vi "Result Step Measure Meter Reading query.vi"(8 "error in (no error)":errorcluster, 10 "Step":T1=1 min=1 max=99 step=1, 11 "VISA resource name":refnum<visa-resource-name>) -> (0 "error out":errorcluster, 2 "Result":string, 3 "VISA resource name out":refnum<visa-resource-name>)   [LabVIEW 2025]
uses:
  <instrlib>/Chroma 19052/Public/Utility/Type Def/steps--numeric.ctl
  <instrlib>/Chroma 19052/Chroma 19052.lvlib
panel:
  # "Step Measure Meter Reading"
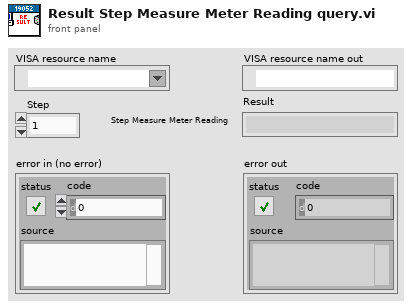
[diagram p1: front panel]
types:
  T1 = typedef "Chroma 19052.lvlib/steps--numeric.ctl" = u8
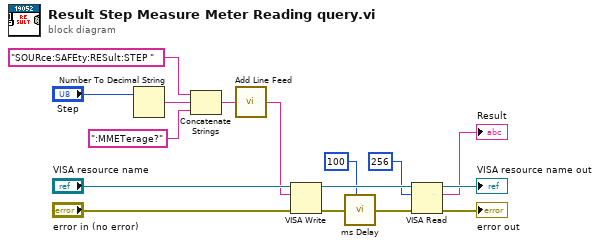
[diagram p0: block diagram]
diagram:
  n1 = Number To Decimal String(number="Step") -> (decimal integer string=w6:string)  [unwired: 1 in]
  n2 = Concatenate Strings("SOURce:SAFEty:RESult:STEP ", w6, ":MMETerage?") -> (w3:string)
  n3 = call <instrlib>:"Add Line Feed.vi"("Command string"=w3) -> ("Concatenated string"=w10:string)  [unwired: 4 in]
  n4 = VISA Write(VISA resource name="VISA resource name", write buffer=w10, error in (no error)="error in (no error)") -> (VISA resource name out=w16:refnum<visa-resource-name>, error out=w15:errorcluster)  [unwired: 1 out]
  n5 = call <instrlib>:"ms Delay.vi"("miliseconds to wait"=u32 100 ("Time Delay ms"), "error in (no error)"=w15) -> ("error out"=w14:errorcluster)  [unwired: 6 in, 1 out]
  n6 = VISA Read(VISA resource name=w16, byte count=u32 256, error in (no error)=w14) -> (VISA resource name out=→"VISA resource name out":refnum<visa-resource-name>, read buffer=→"Result":string, error out=→"error out":errorcluster)  [unwired: 1 out]
